vi "UI NE-500.vi"(8 "error in":errorcluster) -> (0 "error out":errorcluster)   [LabVIEW 2019, in "NE-500.lvlib"]
uses:
  NE-500.lvlib
  User Event/Controls/UE Abort Action.ctl
  <vilib>/Utility/miscctls.llb/LVPointTypeDef.ctl
  Queues/Queues.lvlib
panel:
  in  "Syringe Pump Control":T1={"Withdraw Rate (ul/min)"=0.0, "Infuse Rate (ul/min)"=0.0, "Direction"=enum."Infuse", "Syringe Diameter(mm)"=13.0, "Syringe Pump Switch"=FALSE}
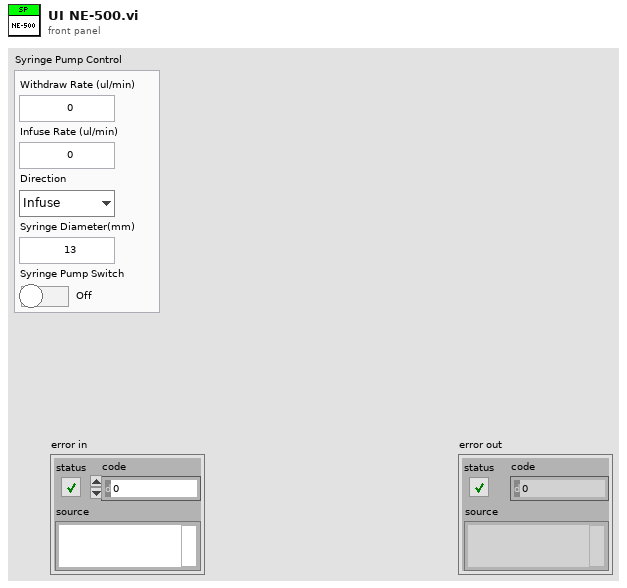
[diagram p1: front panel]
types:
  T1 = cluster{"Withdraw Rate (ul/min)":dbl, "Infuse Rate (ul/min)":dbl, "Direction":enum16{"Infuse", "Withdraw"}, "Syringe Diameter(mm)":dbl, "Syringe Pump Switch":bool}
  T2 = typedef "UE Abort Action.ctl" = enum16{"Create", "Get", "Destroy"}
  T3 = typedef "LVPointTypeDef.ctl" = cluster{"Horizontal":i16, "Vertical":i16}
  T4 = enum16{"Open Pump", "Read", "Set", "Run", "Stop", "Close Pump"}
  T5 = cluster{"Wdr Rate(UM)":dbl, "Inf Rate(UM)":dbl, "Dir":enum16{"Infuse", "Withdraw"}, "Dia(mm)":dbl}
  T6 = typedef "NE-500.lvlib/SEQ Data.ctl" = cluster{"Status":string, "Initialize Done?":bool, "VI Refnum":refnum<vi>}
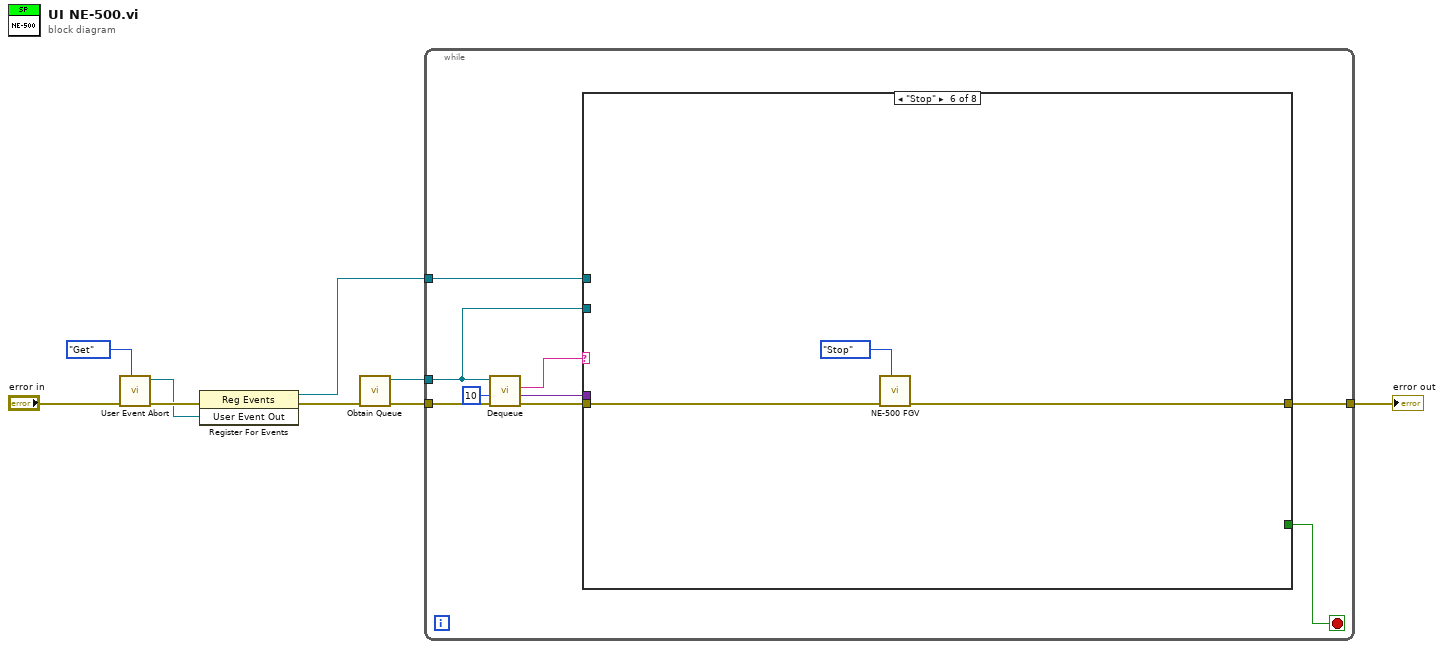
[diagram p0: block diagram]
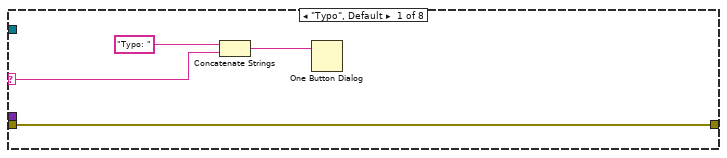
[diagram p2: hidden frame]
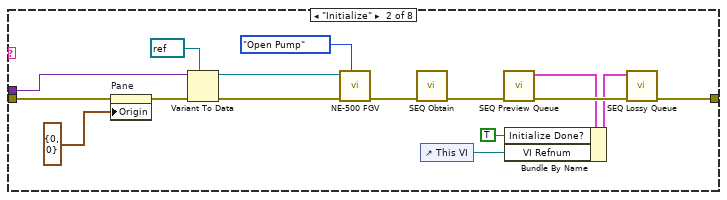
[diagram p3: hidden frame]
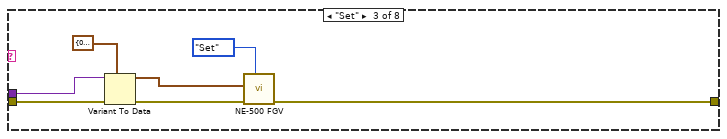
[diagram p4: hidden frame]
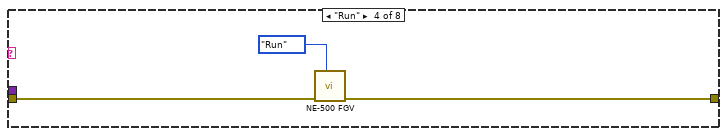
[diagram p5: hidden frame]
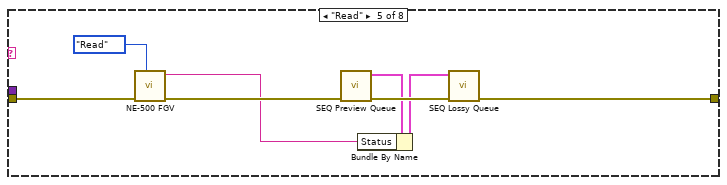
[diagram p6: hidden frame]
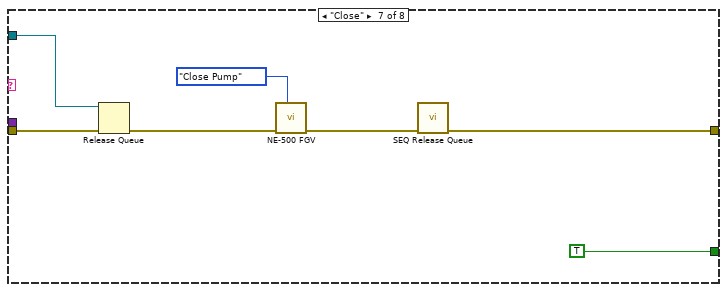
[diagram p7: hidden frame]
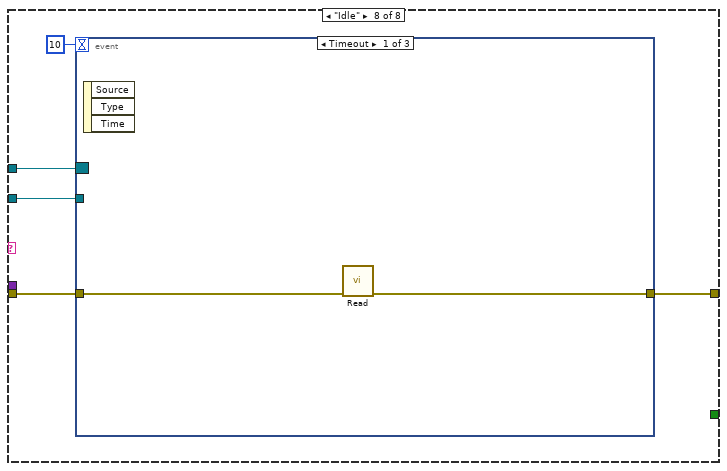
[diagram p8: hidden frame]
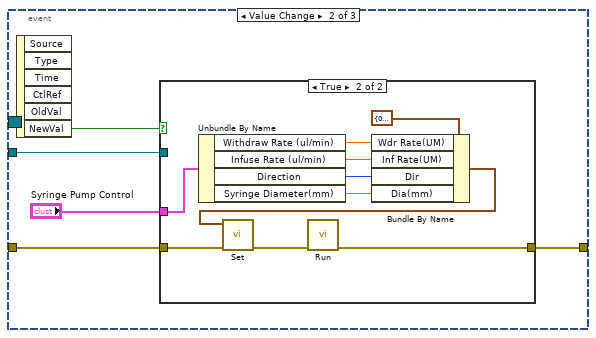
[diagram p9: hidden frame]
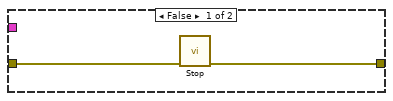
[diagram p10: hidden frame]
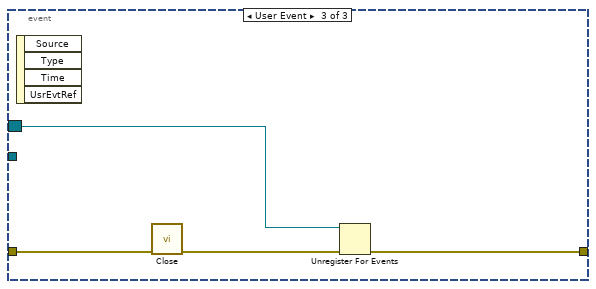
[diagram p11: hidden frame]
diagram:
  n1 = call "User Event Abort.vi"("Action"=UE_Abort_Action."Get", "Error In"="error in") -> ("Error Out"=w7:errorcluster, "User Event Out"=w6:refnum<user-event>)  [unwired: 8 in]
  n2 = register-events(error in=w7, w6) -> (reference out=w4:refnum<event-registration>, error out=w3:errorcluster)  [unwired: 1 in]
  n3 = call "Obtain Queue.vi"("Error In"=w3) -> ("Error Out"=w2:errorcluster, "Queue out"=w1:refnum<queue>)  [unwired: 9 in]
  n4 = while {
    tunnel: w2 -> [w18]
    tunnel: w1 -> [w13]
    tunnel: [w12] -> w5
    tunnel: w4 -> [w11]
    stop <- w10 stop-if-true
    n5 = call "Dequeue.vi"("Error In"=w18, "timeout in ms (-1)"=10, "Queue in"=w13) -> ("Error Out"=w17:errorcluster, "Data"=w15:variant, "State"=w16:string)  [unwired: 5 in, 1 out]
    n6 = case shown="\"Stop\"" w16 {
      selector: w16 -> [w19 _ _ _ _ _ _ _]
      tunnel: w17 -> [w22 w26 w45 w48 w56 w57 w66 w70]
      tunnel: w15 -> [_ w36 w44 _ _ _ _ _]
      tunnel: w13 -> [_ _ _ _ _ _ w65 w67]
      tunnel: [w22 w32 w41 w47 w49 w59 w60 w69] -> w12
      tunnel: w11 -> [_ _ _ _ _ _ _ w68]
      tunnel: [_ _ _ _ _ _ TRUE _] -> w10
      frame "Typo", Default {
        n7 = Concatenate Strings("Typo: " ("string"), w19) -> (w21:string)
        n8 = One Button Dialog(message=w21) -> ()  [unwired: 1 in, 1 out]
      }
      frame "Initialize" {
        n9 = property on="Pane" class="Pane"(error in=w26, "Origin"=T3 {"Horizontal"=0, "Vertical"=0}) -> (error out=w25:errorcluster)  [unwired: 1 in, 1 out]
        n10 = Variant To Data(error in=w25, type=refnum<visa-resource-name> refnum ("VISA resource"), Variant=w36) -> (data=w35:refnum<visa-resource-name>, error out=w38:errorcluster)
        n11 = call "NE-500 FGV.vi"("Function"=T4."Open Pump", "error in"=w38, "VISA resource"=w35) -> ("error out"=w28:errorcluster)  [unwired: 7 in, 1 out]
        n12 = call "SEQ Obtain.vi"("error in"=w28) -> ("error out"=w27:errorcluster)  [unwired: 9 in, 1 out]
        n13 = control-ref of="This VI"() -> (w23:refnum<vi>)
        n14 = call "SEQ Preview Queue.vi"("error in"=w27) -> ("error out"=w33:errorcluster, "SEQ Data"=w31:T6)  [unwired: 9 in]
        n15 = Bundle By Name(cluster=w31, "Initialize Done?"=TRUE, "VI Refnum"=w23) -> (w30:T6)
        n16 = call "SEQ Lossy Queue.vi"("error in"=w33, "SEQ Data"=w30) -> ("error out"=w32:errorcluster)  [unwired: 9 in]
      }
      frame "Set" {
        n17 = Variant To Data(error in=w45, type=T5 {"Wdr Rate(UM)"=0.0, "Inf Rate(UM)"=0.0, "Dir"=enum."Infuse", "Dia(mm)"=0.0} ("Setting"), Variant=w44) -> (data=w40:T5, error out=w42:errorcluster)
        n18 = call "NE-500 FGV.vi"("Function"=T4."Set", "error in"=w42, "Setting"=w40) -> ("error out"=w41:errorcluster)  [unwired: 7 in, 1 out]
      }
      frame "Run" {
        n19 = call "NE-500 FGV.vi"("Function"=T4."Run", "error in"=w48) -> ("error out"=w47:errorcluster)  [unwired: 8 in, 1 out]
      }
      frame "Read" {
        n20 = call "NE-500 FGV.vi"("Function"=T4."Read", "error in"=w56) -> ("error out"=w54:errorcluster, "Read String"=w50:string)  [unwired: 8 in]
        n21 = call "SEQ Preview Queue.vi"("error in"=w54) -> ("error out"=w53:errorcluster, "SEQ Data"=w52:T6)  [unwired: 9 in]
        n22 = Bundle By Name(cluster=w52, "Status"=w50) -> (w51:T6)
        n23 = call "SEQ Lossy Queue.vi"("error in"=w53, "SEQ Data"=w51) -> ("error out"=w49:errorcluster)  [unwired: 9 in]
      }
      frame "Stop" {
        n24 = call "NE-500 FGV.vi"("Function"=T4."Stop", "error in"=w57) -> ("error out"=w59:errorcluster)  [unwired: 8 in, 1 out]
      }
      frame "Close" {
        n25 = Release Queue(queue=w65, error in (no error)=w66) -> (error out=w63:errorcluster)  [unwired: 1 in, 2 out]
        n26 = call "NE-500 FGV.vi"("Function"=T4."Close Pump", "error in"=w63) -> ("error out"=w61:errorcluster)  [unwired: 8 in, 1 out]
        n27 = call "SEQ Release Queue.vi"("error in"=w61) -> ("error out"=w60:errorcluster)  [unwired: 10 in]
      }
      frame "Idle" {
        n28 = event shown="[0] Timeout" {
          selector: w68 -> [_ _ w94]
          dyn-events: _ -> [_ _ _]
          timeout: 10 -> [_ _ _]
          tunnel: w70 -> [w73 w78 w92]
          tunnel: [w72 w76 w93] -> w69
          tunnel: w67 -> [_ w74 _]
          event Timeout {
            n29 = event-data() -> ()  [unwired: 1 in, 3 out]
            n30 = call "Read.vi"("Error In"=w73) -> ("Error Out"=w72:errorcluster)  [unwired: 10 in]
          }
          event "Syringe Pump Control.Syringe Pump Switch": Value Change {
            n31 = event-data() -> ("NewVal"=w77:bool)  [unwired: 1 in, 5 out]
            n32 = case shown="True" w77 {
              tunnel: w78 -> [w79 w90]
              tunnel: [w80 w81] -> w76
              tunnel: "Syringe Pump Control" -> [_ w88]
              tunnel: w74 -> [_ _]
              frame False {
                n33 = call "Stop.vi"("Error In"=w79) -> ("Error Out"=w80:errorcluster)  [unwired: 10 in]
              }
              frame True {
                n34 = Unbundle By Name(w88) -> ("Withdraw Rate (ul/min)"=w86:dbl, "Infuse Rate (ul/min)"=w85:dbl, "Direction"=w84:enum16{"Infuse", "Withdraw"}, "Syringe Diameter(mm)"=w83:dbl)
                n35 = Bundle By Name(cluster=T5 {"Wdr Rate(UM)"=0.0, "Inf Rate(UM)"=0.0, "Dir"=enum."Infuse", "Dia(mm)"=0.0} ("Setting"), "Wdr Rate(UM)"=w86, "Inf Rate(UM)"=w85, "Dir"=w84, "Dia(mm)"=w83) -> (w82:T5)
                n36 = call "Set.vi"("Error In"=w90, "Setting"=w82) -> ("Error Out"=w89:errorcluster)  [unwired: 9 in]
                n37 = call "Run.vi"("Error In"=w89) -> ("Error Out"=w81:errorcluster)  [unwired: 10 in]
              }
            }
          }
          event User Event {
            n38 = event-data() -> ()  [unwired: 1 in, 4 out]
            n39 = call "Close.vi"("Error In"=w92) -> ("Error Out"=w91:errorcluster)  [unwired: 10 in]
            n40 = Unregister For Events(event registration refnum=w94, error in=w91) -> (error out=w93:errorcluster)
          }
        }
      }
    }
  }
  "error out" <- w5
